vi "getTopicTypesReply.vi"(3 "ROS_Master.lvclass in":refnum<class "ROS_Master.lvclass">) -> (1 "Topics XML":string)   [LabVIEW 2013, in "ROS_Master.lvclass"]
uses:
  <userlib>/ROSforLV/ROS/Code/SubVIs/ROS_Master/ROS_Master.lvclass
  <userlib>/ROSforLV/ROS/Code/SubVIs/ROS_Master/ROS_Master.lvclass/ROS_Master.ctl
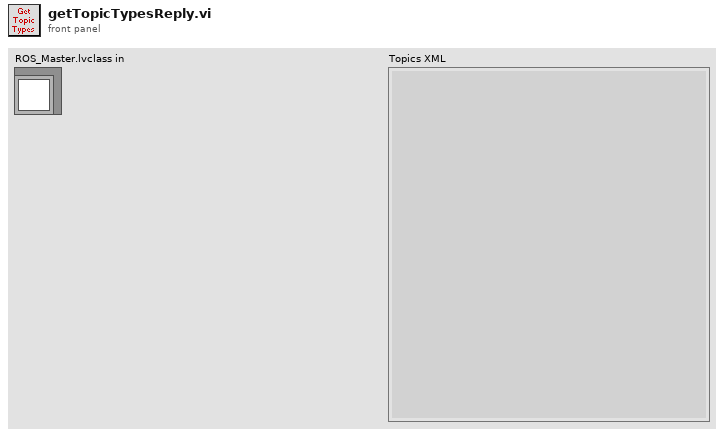
[diagram p1: front panel]
types:
  T1 = cluster{"Name":string, "PubSubs":cluster{"Caller ID":string, "IP":string, "Msg Type":string, "Direction":enum16{"Publisher", "Subscriber"}, "Topic":string}[]}[]
  T2 = cluster{"Caller ID":string, "IP":string, "Msg Type":string, "Direction":enum16{"Publisher", "Subscriber"}, "Topic":string}[]
  T3 = cluster{"Caller ID":string, "IP":string, "Msg Type":string, "Direction":enum16{"Publisher", "Subscriber"}, "Topic":string}
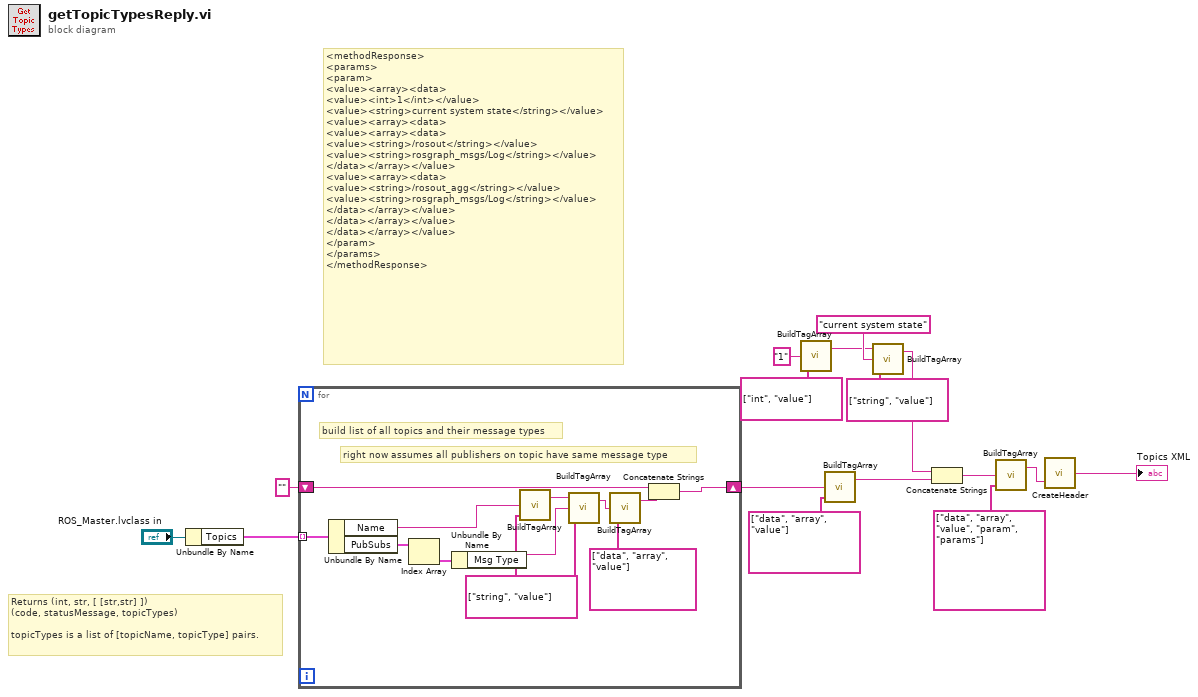
[diagram p0: block diagram]
diagram:
  # "<methodResponse>\n<params>\n<param>\n<value><array><data>\n<value><int>1</int></value>\n<value><string>current system state</string></value>\n<value><array><data>\n<value><array><data>\n<value><string>/rosout</string></value>\n<value><string>rosgraph_msgs/Log</string></value>\n</data></array></value>\n<value><array><data>\n<value><string>/rosout_agg</string></value>\n<value><string>rosgraph_msgs/Log</string></value>\n</data></array></value>\n</data></array></value>\n</data></array></value>\n</param>\n</params>\n</methodResponse>"
  # "Returns (int, str, [ [str,str] ])\n(code, statusMessage, topicTypes)\n\ntopicTypes is a list of [topicName, topicType] pairs."
  n1 = Unbundle By Name("ROS_Master.lvclass in") -> ("Topics"=w1:T1)
  n2 = for {
    tunnel: w1 -> [w28] mode=indexing
    shift-right: [w26] -> w8
    shift-left: "" ("string out") -> [w27]
    w21 = string[] ["string", "value"] ("tags")
    # "right now assumes all publishers on topic have same message type"
    # "build list of all topics and their message types"
    n3 = Unbundle By Name(w28) -> ("Name"=w25:string, "PubSubs"=w24:T2)
    n4 = Index Array(array=w24) -> (element=w23:T3)  [unwired: 1 in]
    n5 = Unbundle By Name(w23) -> ("Msg Type"=w17:string)
    n6 = call <userlib>:"BuildTagArray.vi"("tags"=w21, "value"=w25) -> ("string out"=w22:string)  [unwired: 2 in]
    n7 = call <userlib>:"BuildTagArray.vi"("tags"=w21, "value"=w17, "string in"=w22) -> ("string out"=w20:string)  [unwired: 1 in]
    n8 = call <userlib>:"BuildTagArray.vi"("tags"=string[] ["data", "array", "value"], "value"=w20) -> ("string out"=w18:string)  [unwired: 2 in]
    n9 = Concatenate Strings(w27, w18) -> (w26:string)
  }
  n10 = call <userlib>:"BuildTagArray.vi"("tags"=string[] ["int", "value"], "value"="1") -> ("string out"=w10:string)  [unwired: 2 in]
  n11 = call <userlib>:"BuildTagArray.vi"("tags"=string[] ["data", "array", "value"], "value"=w8) -> ("string out"=w7:string)  [unwired: 2 in]
  n12 = call <userlib>:"BuildTagArray.vi"("tags"=string[] ["string", "value"], "value"="current system state", "string in"=w10) -> ("string out"=w9:string)  [unwired: 1 in]
  n13 = Concatenate Strings(w9, w7) -> (w6:string)
  n14 = call <userlib>:"BuildTagArray.vi"("tags"=string[] ["data", "array", "value", "param", "params"], "value"=w6) -> ("string out"=w3:string)  [unwired: 2 in]
  n15 = call <userlib>:"CreateHeader.vi"("Content"=w3) -> ("XML"=→"Topics XML":string)  [unwired: 1 in]
